vi "ExceptionStatus.vi"(8 "错误输入（无错误）":errorcluster, 9 "SocketQueue":T1, 10 "connection ID输入":refnum<k5>, 11 "socket 2":T2={"端口"=10013, "timeout"=10013, "标准差倍数"=0.0, "address"="{\"ad\":1}", "normal"="{\"ad\":0}"}) -> (0 "错误输出":errorcluster, 1 "connection ID输出":refnum<k5>)   [LabVIEW 2018]
uses:
  Initialize/Setting/SocketData.ctl
  Initialize/CreateQueue/SocketQueue.ctl
  <vilib>/Analysis/baseanly.llb/Mean (DBL).vi
  <vilib>/Analysis/NI_AALBase.lvlib
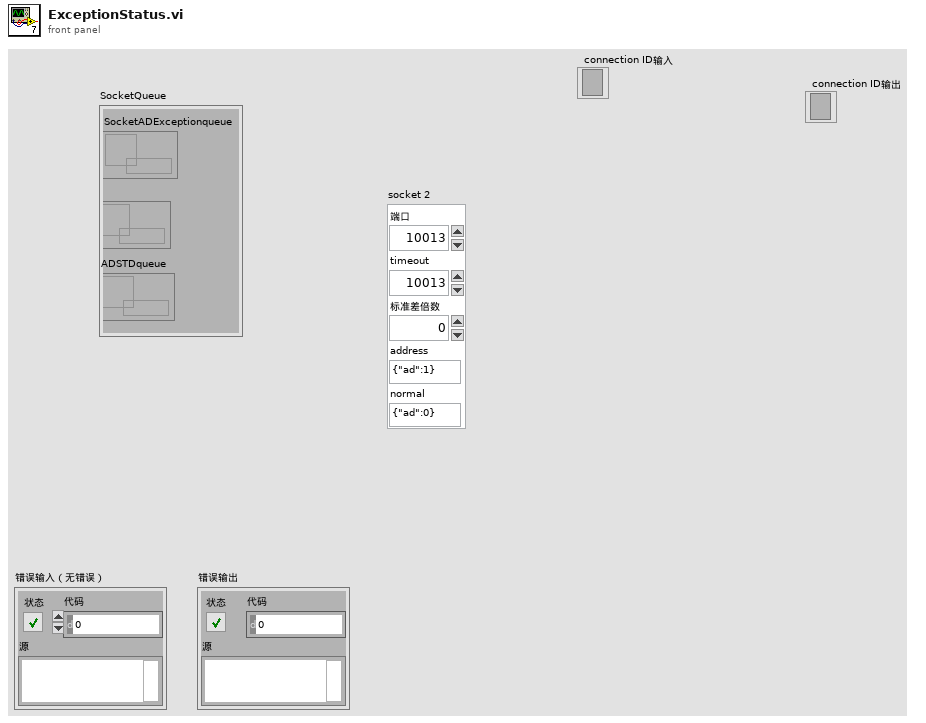
[diagram p1: front panel]
types:
  T1 = typedef "SocketQueue.ctl" = cluster{"ADSTDqueue ":refnum<queue>, "SocketADExceptionqueue":refnum<queue>, "  SocketAD":refnum<queue>}
  T2 = typedef "SocketData.ctl" = cluster{"端口":u16, "timeout":u16, "标准差倍数":dbl, "address":string, "normal":string}
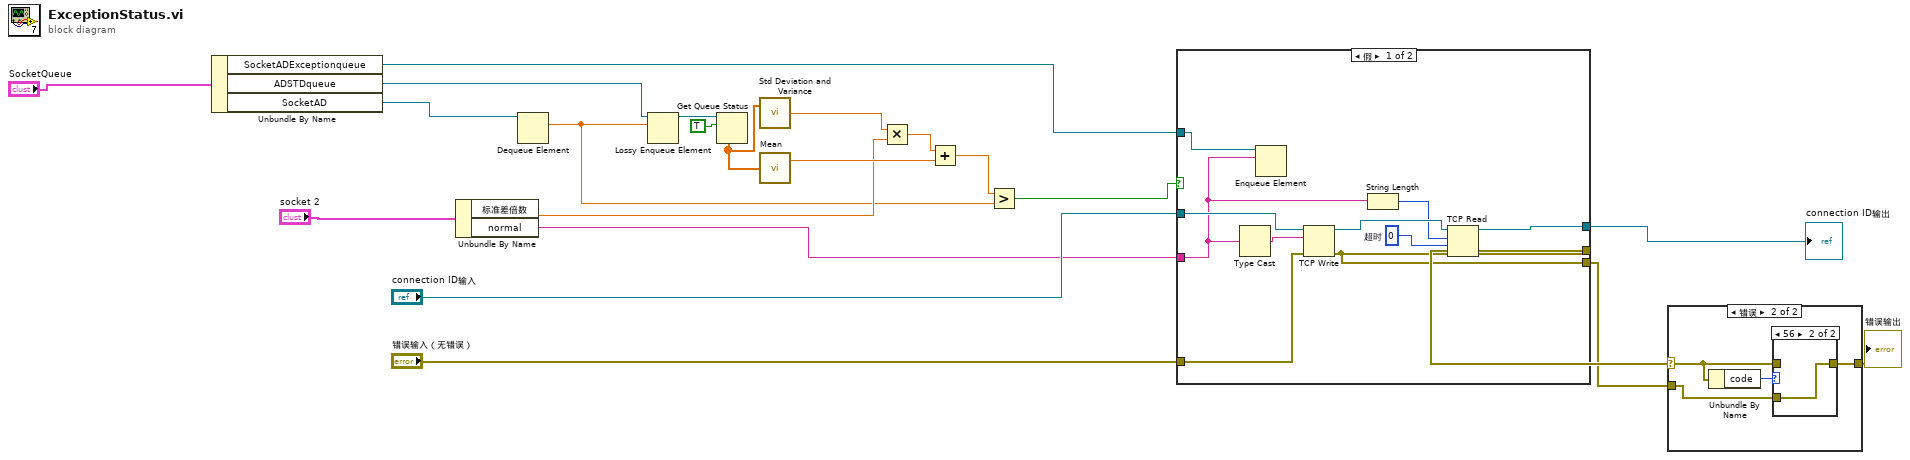
[diagram p0: block diagram]
diagram:
  n1 = Unbundle By Name("SocketQueue") -> ("SocketADExceptionqueue"=w7:refnum<queue>, "ADSTDqueue"=w12:refnum<queue>, "SocketAD"=w6:refnum<queue>)
  n2 = Unbundle By Name("socket 2") -> ("标准差倍数"=w4:dbl, "normal"=w9:string)
  n3 = Dequeue Element(queue=w6) -> (element=w2:dbl)  [unwired: 2 in, 3 out]
  n4 = Lossy Enqueue Element(queue=w12, element=w2) -> (queue out=w13:refnum<queue>)  [unwired: 1 in, 3 out]
  n5 = Get Queue Status(queue=w13, return elements? (F)=TRUE ("返回元素？(F)")) -> (elements=w11:dbl[])  [unwired: 1 in, 7 out]
  n6 = call <vilib>:"Std Deviation and Variance.vi"("X"=w11) -> ("standard deviation"=w5:dbl)  [unwired: 1 in, 2 out]
  n7 = call-poly <vilib>:"Mean.vi"("X"=w11) -> ("mean"=w10:dbl)  [unwired: 1 out]
  n8 = Multiply(x=w5, y=w4) -> (x*y=w14:dbl)
  n9 = Add(x=w14, y=w10) -> (x+y=w3:dbl)
  n10 = Greater?(x=w3, y=w2) -> (0:w22:bool)
  n11 = case shown="假" w22 {
    tunnel: "connection ID输入" -> [w29 _]
    tunnel: [w28 _] -> w19
    tunnel: [w26 _] -> w21
    tunnel: [w27 _] -> w18
    tunnel: "错误输入（无错误）" -> [w30 _]
    tunnel: w7 -> [w25 _]
    tunnel: w9 -> [w24 _]
    frame False {
      w33 = 0  # 超时
      n12 = Type Cast(x=w24) -> (*(type *) &x=w32:string)  [unwired: 1 out]
      n13 = Enqueue Element(queue=w25, element=w24) -> ()  [unwired: 2 in, 3 out]
      n14 = TCP Write(connection ID=w29, data in=w32, error in (no error)=w30) -> (connection ID out=w31:refnum<k5>, error out=w27:errorcluster)  [unwired: 2 out]
      n15 = String Length(string=w24) -> (length=w23:i32)
      n16 = TCP Read(connection ID=w31, bytes to read=w23, error in (no error)=w27, 9:w33) -> (connection ID out=w26:refnum<k5>, error out=w28:errorcluster)  [unwired: 1 in, 1 out]
    }
    frame True {
    }
  }
  "connection ID输出" <- w21
  n17 = case shown="错误" w19 {
    selector: w19 -> [w34 w37]
    tunnel: [w34 w35] -> w20
    tunnel: w18 -> [_ w36]
    frame No Error {
    }
    frame Error {
      n18 = Unbundle By Name(w37) -> ("code"=w38:i32)
      n19 = case shown="56" w38 {
        tunnel: w37 -> [w39 _]
        tunnel: w36 -> [_ w40]
        tunnel: [w39 w40] -> w35
        frame Default {
        }
        frame 56 {
        }
      }
    }
  }
  "错误输出" <- w20
